vi "Testing Mode.vi"(7 "Filepath":path=path "D:/My Project/2019-2020/Magnetic Mareli UM/MM_UM/Project Setup/data/program seq/Program_280A.bin") -> (1 "Running Model":string)   [LabVIEW 2015]
uses:
  Control Button/Exit.ctl
  Control Button/Start.ctl
  Test  enqueue/AutoTest seq.ctl
  Test  enqueue/Auot Test selection.ctl
  <vilib>/Analysis/baseanly.llb/Mean (DBL).vi
  Galobal variable_TI.vi
  Project Setup/Globle Variable/GR_Servo.vi
  <vilib>/Utility/file.llb/Read Delimited Spreadsheet (string).vi
  <vilib>/Utility/file.llb/Write Delimited Spreadsheet (string).vi
  <vilib>/Analysis/NI_AALBase.lvlib
panel:
  out "Error code":string
  out "Camera Status":T1
  out "x .and. y?":bool
  out "Error":bool
  in  "value":bool
  in  "Tracibility":bool=TRUE
  out "In Range?":bool
  in  "Result":string
  out "Barcode Setting":T2
  in  "Total Counter":string
  out "D.S Tail Tell Barcode":string
  out "D.S Blinker Barcode":string
  out "Dail Speedo Barcode":string
  out "Reset":bool
  out "Emergency":bool
  out "Max Load(N)":string
  out "Min Load(N)":string
  in  "Actual Load(N)":string
  out "Load Cell":dbl format="%0.03f"
  in  "Load Offset":dbl
  out "max value":dbl
  out "Dail RPM Barcode":string
  out "Camera NG_P13":bool
  out "Camera OK_P12":bool
  out "Difusser_AI5":bool
  out "Difusser_AI4":bool
  out "Job ID":string
  in  "Graph Reset":bool
  in  "Safety Enb":bool
  in  "Tab Control":enum32{"Test", "Home call"}(tab)
  in  "test":string[][](table)=[["1", "Light Box Ionization", "Pass"], ["2", "Light box Clamp", "Pass"], ["3", "Difusser Put on Light Box", "Pass"], ["4", "Photo Prism Put On LB", "Test In Progress"], ["5", "LCD Put On Light Box", ""], ["6", "Difusser Checking Position", ""], ["7", "Adesive Tap check Camera", ""], ["8", "LCD Placing Position", ""], ["9", "Camera check Adhesive Taps", ""], ["10", "LCD Display Rotating ", ""], ["11", "Camera Slide Unit", ""], ["12", "LCD Pressing Servo", ""], ["13", "LCD Pressing servo up", ""], ["14", "Camera Unit Rev", ""], ["15", "Fixture Slide Up", ""], ["16", "Light Box Unclamp", ""]]
  in  "Home":string[][](table)
  out "stripped path":path
  in  "Tab":enum32{"Image Display", "Load Graph"}(tab)
  out "2D Picture":picture
  out "Force Vs Time":dbl[](graph)
  in  "String":string
  in  "Vacuum bit":bool
  out "MIC Code":string
  out "Date time":string
  in  "NG Counter":string
  in  "OK Counter":string
  out "User Name":string
  in  "Cycle":i32
  in  "Slide Servo Home Call":bool
  out "D-enqueue":T3
  in  "Home Call":bool
  out "DI":bool[](array[boolean])
  in  "Error Message":string
  out "Current Date & Time":timestamp
  out "Cycle Time(Sec)":i32
  in  "Start":T4
  in  "Cycle Start Bit":bool
  in  "vi reference":refnum<vi>
  in  "Reset Ct.":bool
  out "error out":errorcluster
  in  "Tbl Refnum":refnum<vi>
  in  "Image Display":bool
  in  "Exit":T5
  # "Enable"
  # "Disable"
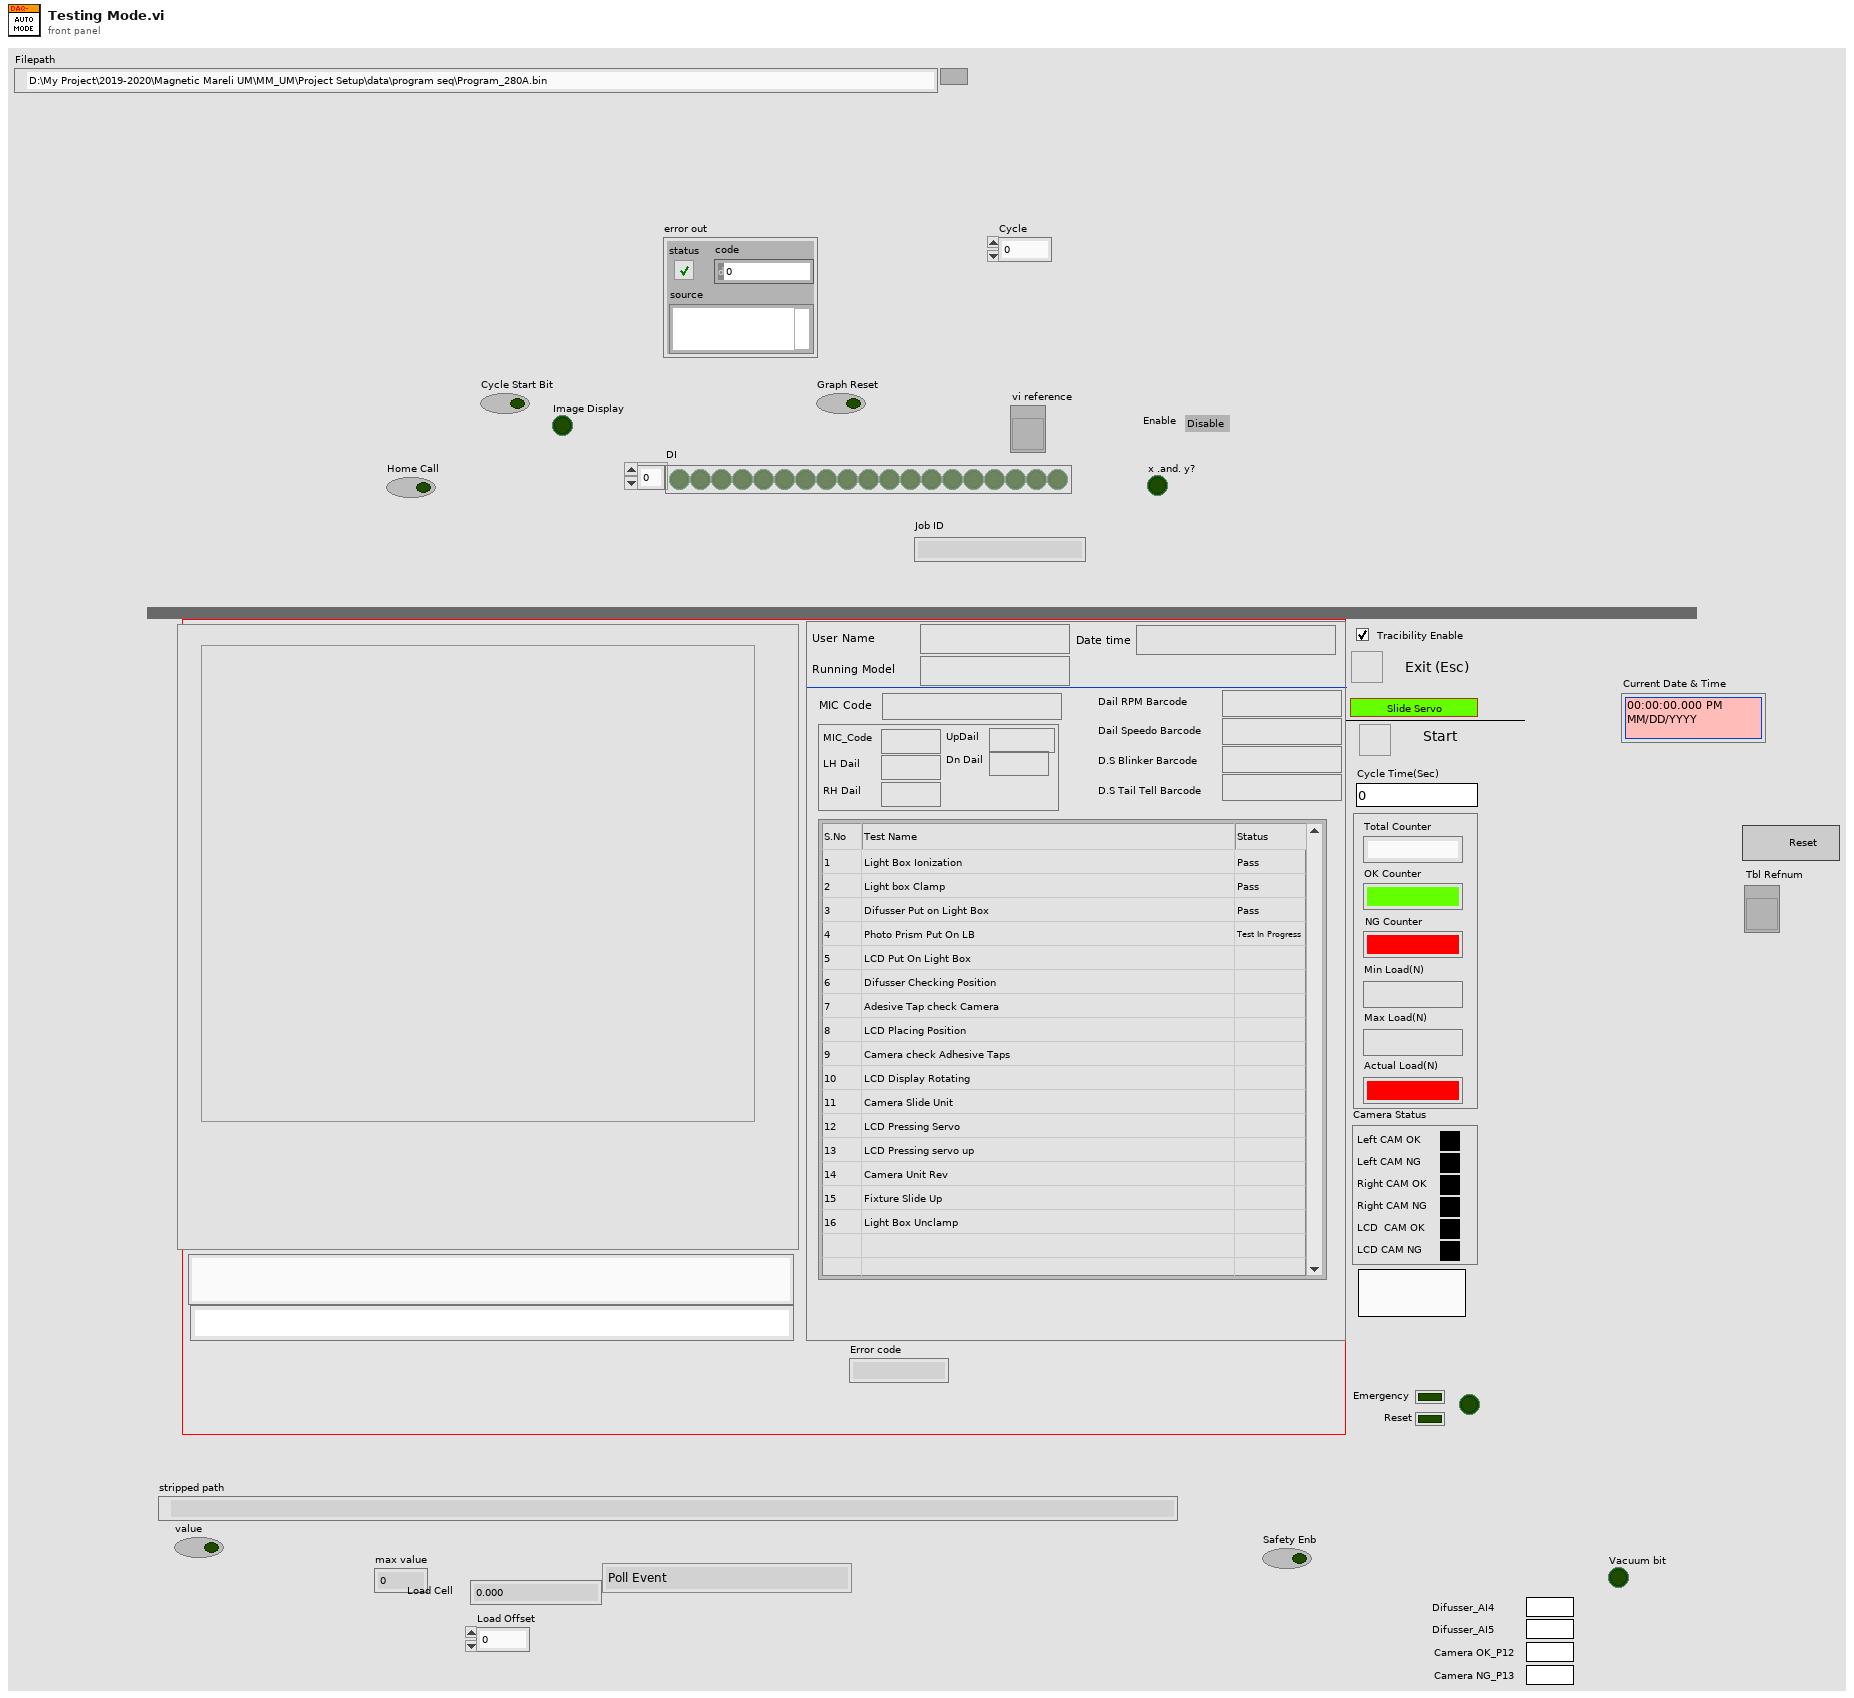
[diagram p1: front panel]
types:
  T1 = cluster{"Left CAM OK":bool, "Left CAM NG":bool, "Right CAM OK":bool, "Right CAM NG":bool, "LCD  CAM OK":bool, "LCD CAM NG ":bool}
  T2 = cluster{"MIC_Code":string, "LH Dail":string, "RH Dail":string, "UpDail":string, "Dn Dail":string}
  T3 = typedef "AutoTest seq.ctl" = enum16{"Poll Event", "Cylender Home ", "Initilization", "Read Barcode", "Slide Servo send Cammand", "Slide Servo Home Call", "Slide Servo Reset", "Camera Co-ordinate_1", "Home Call", "Result Save", "Exit"}
  T4 = typedef "Start.ctl" = bool
  T5 = typedef "Exit.ctl" = bool
  T6 = typedef "Auot Test selection.ctl" = enum16{"Init", "Enqueue ", "Enqueue N", "Enqueue in stack", "Enqueue in stack N", "Dequeue", "Dequeue N", "Flush", "Release Queue"}
  T7 = cluster{"MaxLoad(N) ":dbl, "Min Load(N)":dbl, "Load Offset":dbl, "Model":string, "MIC Code":string, "Dial Speedo":string, "Dial RMP":string, "Blinker":string, "Telltale":string}
  T8 = cluster{"Item Name":string, "Item Status":bool, "Steps":cluster{"Channel Type":string, "Channels":string, "Wait/Poll (ms)":u32, "Parameter":u8, "STM-Speed":i32, "STM-Degree":u32, "Direction":u8}[]}[]
  T9 = cluster{"No. Fail Coun t":string, "Rework Status Count 0\\1":string, "NA Count Max =3 ":string, "Testesd Count  0/1":string, "Error code":string}
  T10 = enum16{"Height Check Cyl up(P0.23_07)", "Height Check Cyl  Up RS_(AI12_26)", "Height Check Cyl  Dn RS_(AI13_27)", "Height Check Cyl dn(P0.24_08)", "Camera Cyl Rev(P0.26_10)", "Camera Cyl fwd(P0.25_09)", "Height Check Cyl off", "Camera Cyl Rev_RS(AI15_29)", "Camera Cyl off", "Camera Cyl FWD_RS(AI14_28)", "LCD Rotation Dn(P0.28_12)", "LCD Rotation dn proxi(AI17_31)", "LCD Rotation Up(P0.27_11)", "LCD Rotation dn proxi(AI16_30)"}
  T11 = cluster{"Start":bool, "Emergency ":bool, "Reset":bool, "Home":bool, "Safety":bool}
  T12 = cluster{"[0]":string, "[1]":string, "[2]":string, "[3]":string, "[4]":string, "[5]":string, "[6]":string, "[7]":string}
  T13 = cluster{"[0]":string, "[1]":string, "[2]":string, "[3]":string, "[4]":string}
  T14 = cluster{"Emergency":bool, "Air Pressure":bool, "Saftey Sensor":bool, "Slide Servo  fault":bool, "Reset":bool, "Pressing Cyl Up RS_AI19":bool}
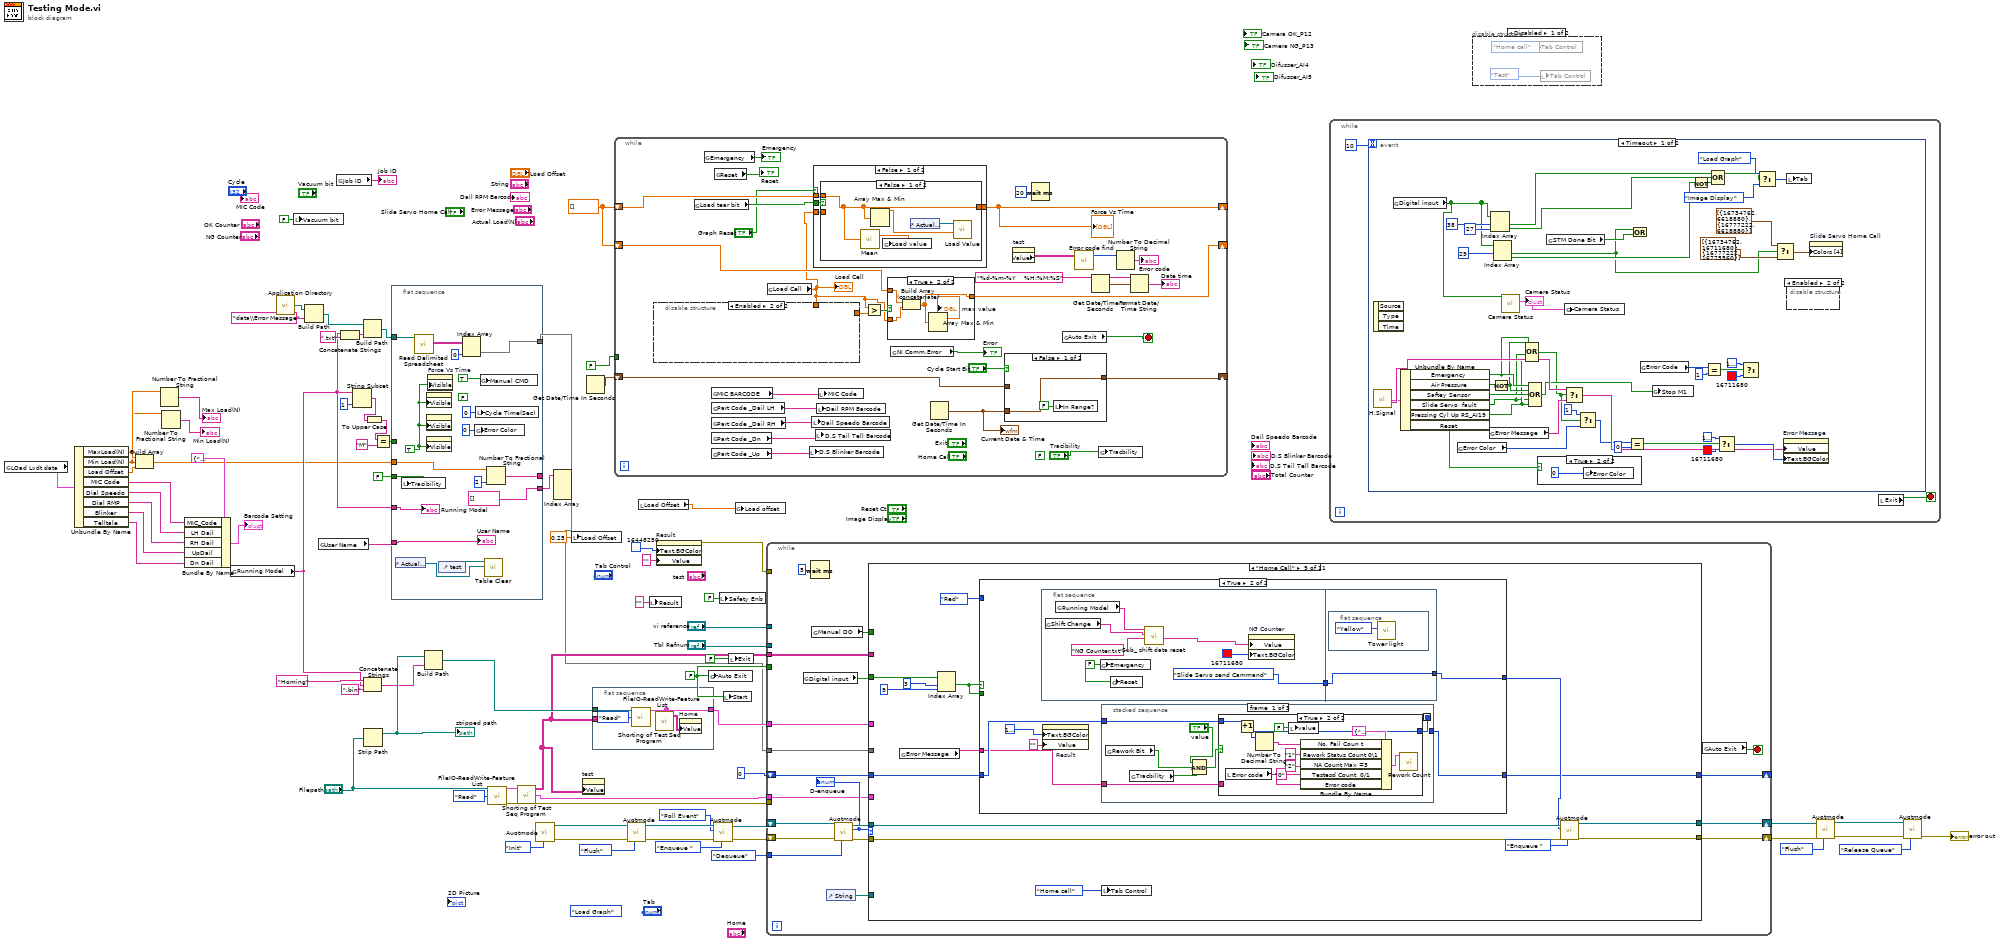
[diagram p0: block diagram]
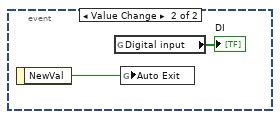
[diagram p5: hidden frame]
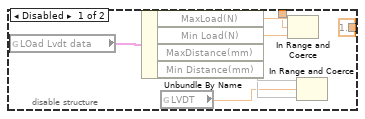
[diagram p6: hidden frame]
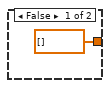
[diagram p7: hidden frame]
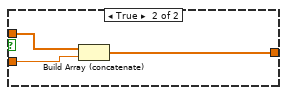
[diagram p8: hidden frame]
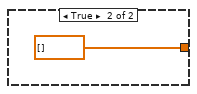
[diagram p9: hidden frame]
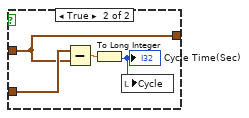
[diagram p10: hidden frame]
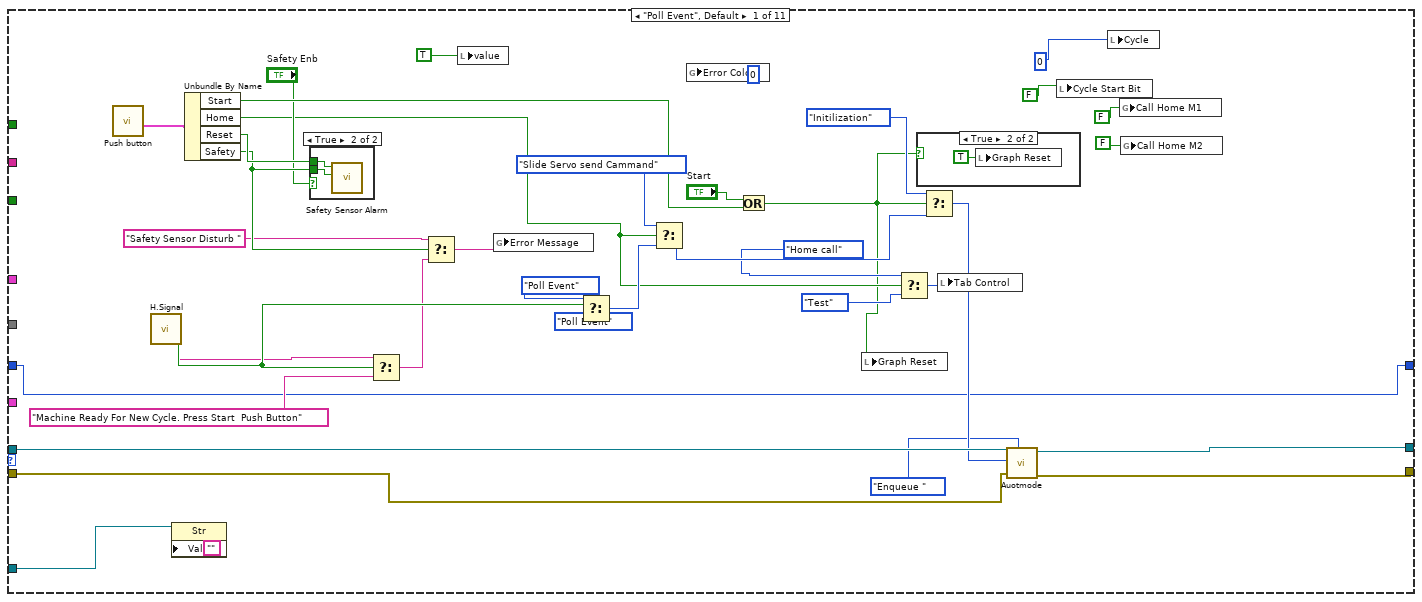
[diagram p11: hidden frame]
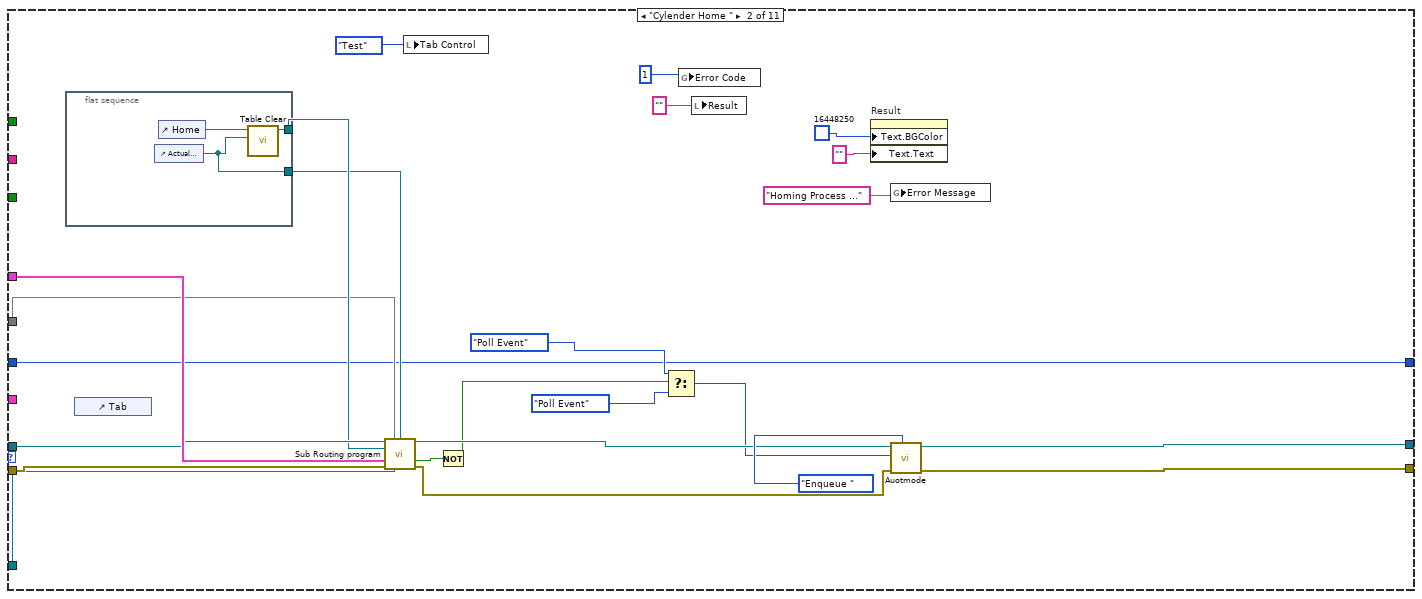
[diagram p14: hidden frame]
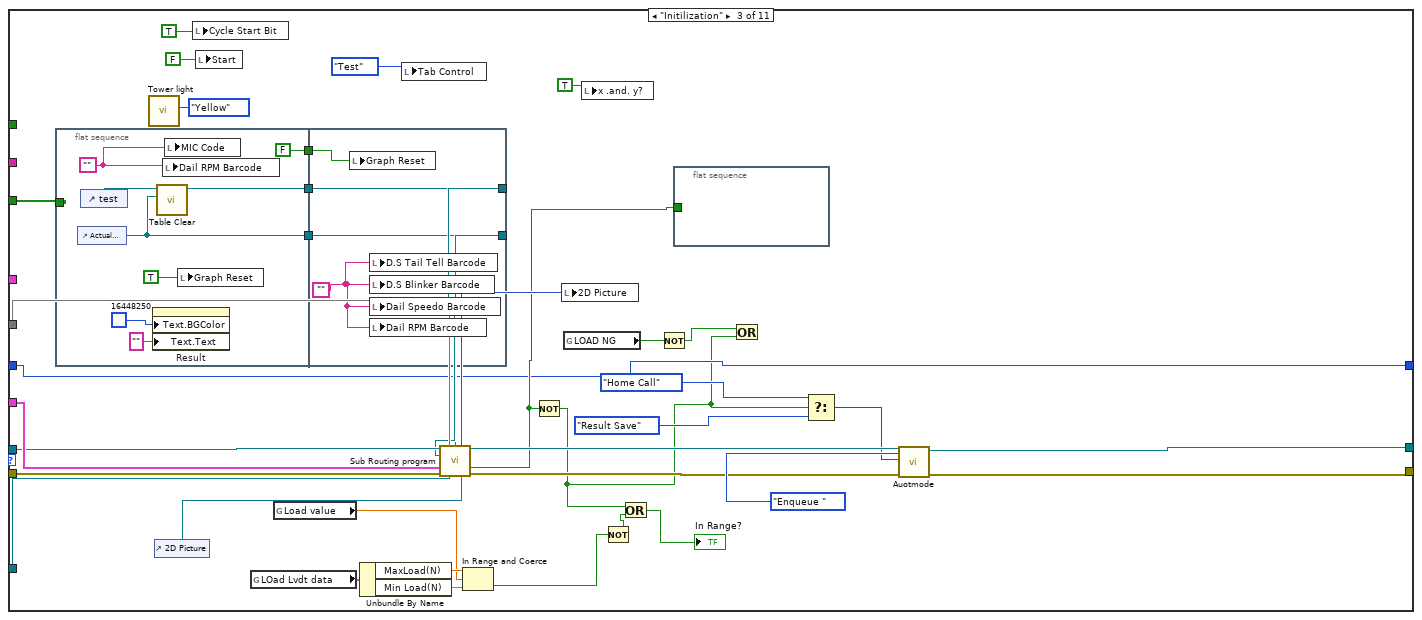
[diagram p15: hidden frame]
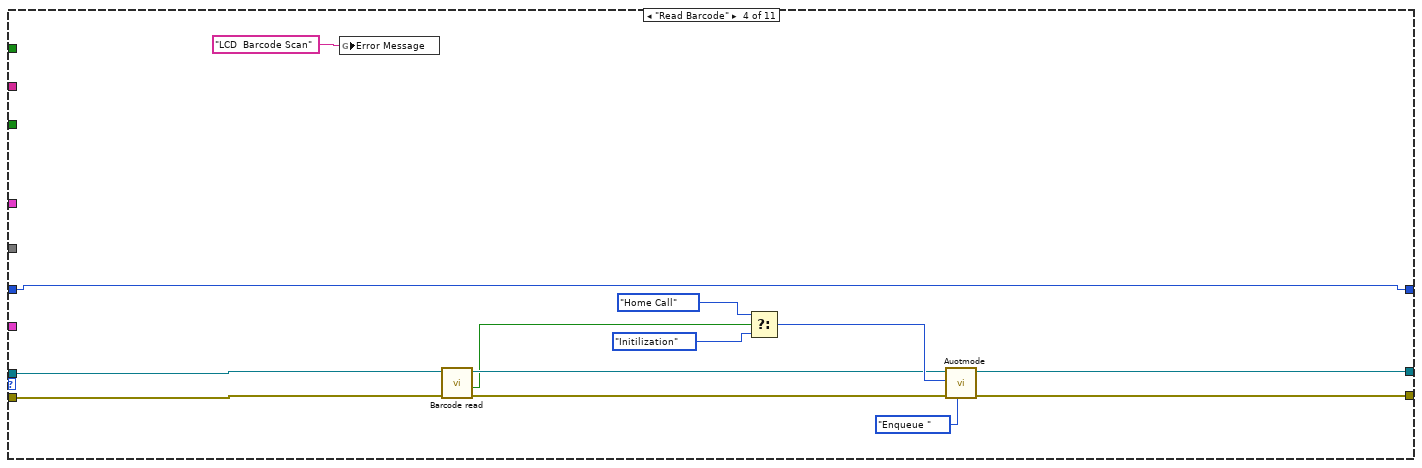
[diagram p16: hidden frame]
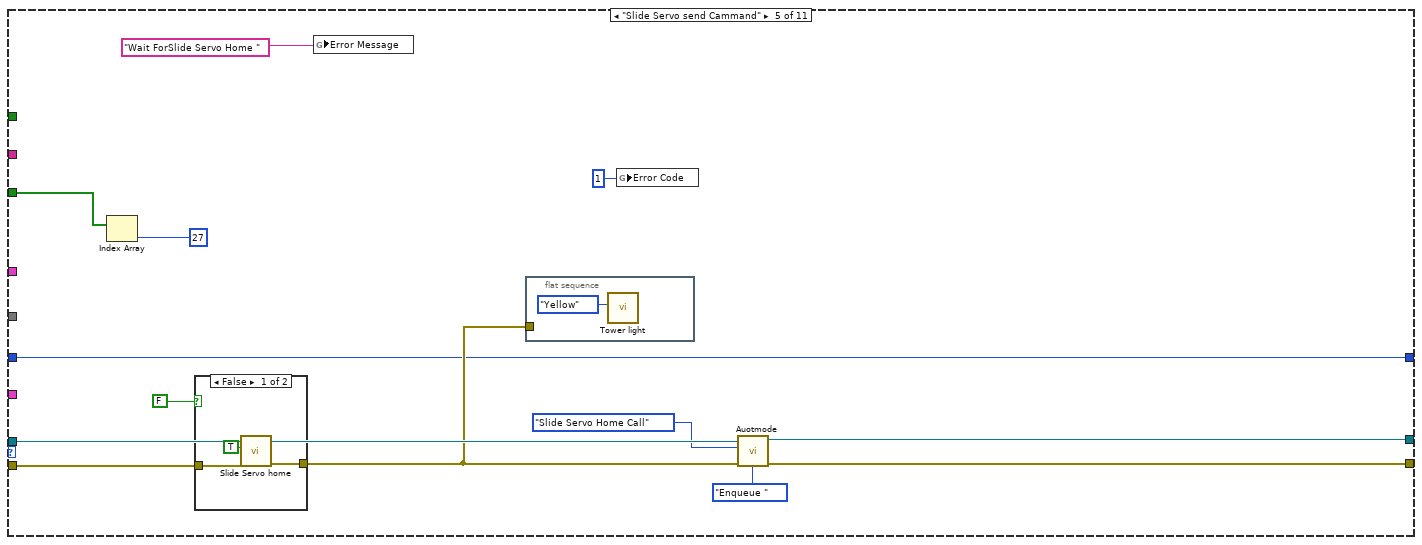
[diagram p17: hidden frame]
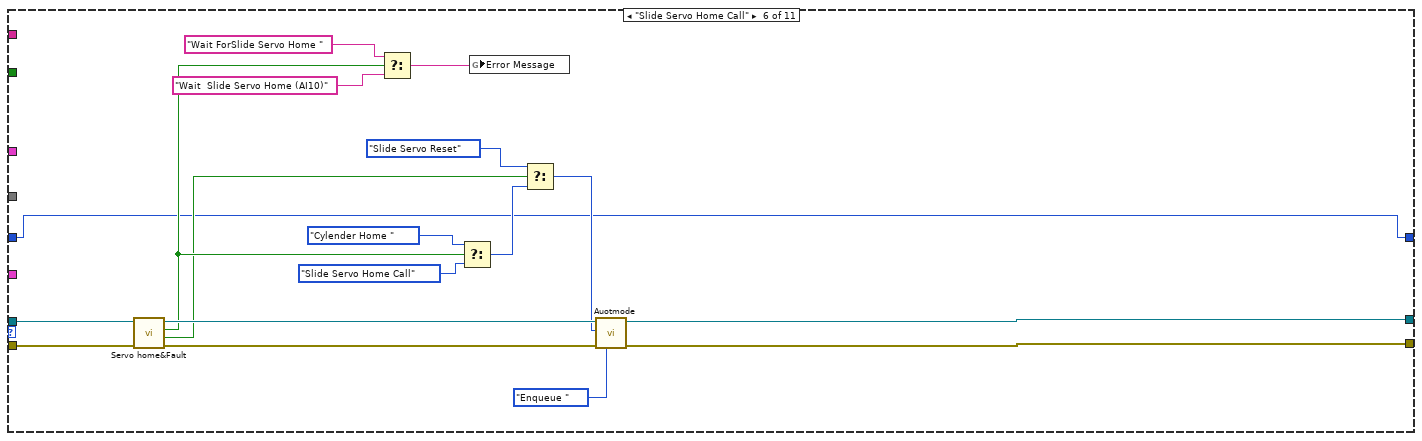
[diagram p19: hidden frame]
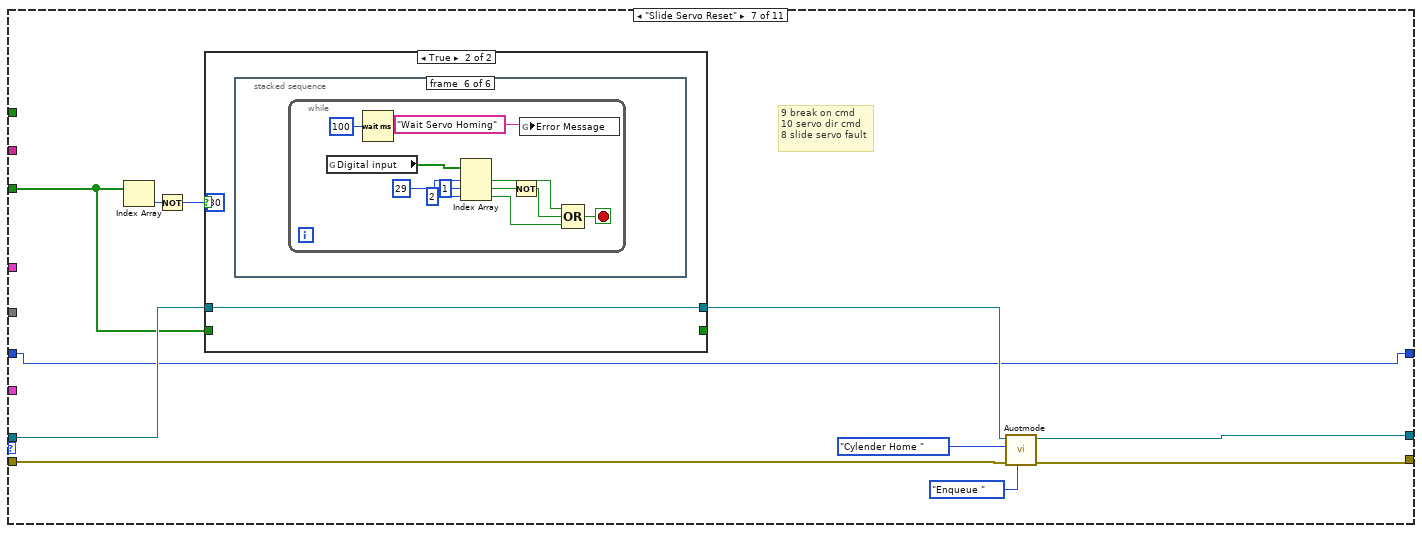
[diagram p20: hidden frame]
diagram:
  (unwired) enum32{"Image Display", "Load Graph"}."Load Graph" ("Tab")
  w41 = dbl[] []
  w53 = FALSE ("Auto Exit")
  n1 = global read "Galobal variable_TI.vi" "LOad Lvdt data"() -> (w22:T7)
  n2 = Unbundle By Name(w22) -> ("MaxLoad(N)"=w8:dbl, "Min Load(N)"=w7:dbl, "Load Offset"=w21:dbl, "MIC Code"=w19:string, "Dial Speedo"=w18:string, "Dial RMP"=w17:string, "Blinker"=w16:string, "Telltale"=w15:string)
  n3 = Build Array(w8, w7, w21) -> (w13:dbl[])
  n4 = Number To Fractional String(number=w8) -> (F-format string=→"Max Load(N)":string)  [unwired: 3 in]
  n5 = Number To Fractional String(number=w7) -> (F-format string=→"Min Load(N)":string)  [unwired: 3 in]
  n6 = Bundle By Name(cluster=T2 {"MIC_Code"="", "LH Dail"="", "RH Dail"="", "UpDail"="", "Dn Dail"=""} ("Barcode Setting"), "MIC_Code"=w19, "LH Dail"=w18, "RH Dail"=w17, "UpDail"=w16, "Dn Dail"=w15) -> (→"Barcode Setting":T2)
  n7 = global read "Galobal variable_TI.vi" "Running Model"() -> (w32:string)
  n8 = call <vilib>:"Application Directory.vi"() -> ("Application Directory"=w37:path)
  n9 = local write "Vacuum bit"(FALSE ("Vacuum bit")) -> ()
  n10 = Build Path(base path=w37, name or relative path="data\\Error Message") -> (appended path=w38:path)
  n11 = global read "Galobal variable_TI.vi" "User Name"() -> (w52:string)
  n12 = global read "Galobal variable_TI.vi" "Job ID"() -> (→"Job ID":string)
  n13 = Concatenate Strings(w32, ".txt" ("string")) -> (w35:string)
  n14 = String Subset(string=w32, length (rest)=1 ("length (rest)")) -> (substring=w27:string)  [unwired: 1 in]
  n15 = Build Path(base path=w38, name or relative path=w35) -> (appended path=w34:path)
  n16 = Concatenate Strings("Homing" ("string"), w32, ".bin" ("string")) -> (w42:string)
  n17 = Strip Path(path="Filepath") -> (stripped path=w49:path)  [unwired: 1 out]
  "stripped path" <- w49
  n18 = To Upper Case(1:w27) -> (0:w30:string)
  n19 = Equal?(x=w30, y="M") -> (x = y?=w28:bool)
  n20 = flat-sequence {
    tunnel: [w92] -> _
    tunnel: w32 -> [w91]
    tunnel: w52 -> [w90]
    tunnel: w34 -> [w87]
    tunnel: [w84] -> w33
    tunnel: w28 -> [_]
    tunnel: [string[] [] ("array")] -> w24
    tunnel: w13 -> [w80]
    tunnel: FALSE -> [w78]
    frame #0 {
      w81 = TRUE
      (unwired) FALSE ("LCD Servo Home Call")
      n21 = control-ref of="Actual Load(N)"() -> (w88:refnum<vi>)
      n22 = local write "Tracibility"(w78) -> ()
      n23 = call-poly <vilib>:"Read Delimited Spreadsheet.vi"("file path (dialog if empty)"=w87) -> ("all rows"=w86:string[][])  [unwired: 9 in, 5 out]
      n24 = property on="Min Load(N)" class="Str"("Visible"=w81) -> ()  [unwired: 2 in, 2 out]
      n25 = property on="Max Load(N)" class="Str"("Visible"=w81) -> ()  [unwired: 2 in, 2 out]
      n26 = property on="Actual Load(N)" class="Str"("Visible"=w81) -> ()  [unwired: 2 in, 2 out]
      n27 = property on="Force Vs Time" class="WFGraph (strict)"("Visible"=w81) -> ()  [unwired: 2 in, 2 out]
      n28 = control-ref of="test"() -> (w89:refnum<vi>)
      n29 = Index Array(array=w86, index (col)=0 ("disabled index (col)")) -> (element=w84:string[])  [unwired: 1 in]
      n30 = global write "GR_Servo.vi" "Error Color"(0 ("Error Color")) -> ()
      n31 = local write "Cycle Time(Sec)"(0 ("Cycle Time(Sec)")) -> ()
      n32 = global write "Galobal variable_TI.vi" "Manual CMD"(TRUE ("Manual CMD")) -> ()
      n33 = call "Table Clear.vi"("Load"=w88, "Table (In)"=w89) -> ()  [unwired: 8 in, 2 out]
      n34 = Number To Fractional String(number=w80, precision (6)=i16 2) -> (F-format string=w92:string[])  [unwired: 2 in]
      "User Name" <- w90
      "Running Model" <- w91
    }
  }
  n35 = Build Path(base path=w49, name or relative path=w42) -> (appended path=w48:path)
  n36 = call "FileIO-ReadWrite-FeatureList.vi"("Filepath"="Filepath", "Read/Write"=enum16{"Read", "Write"}."Read") -> ("Feature List (Out)"=w58:T8, "Error Out"=w59:errorcluster)  [unwired: 12 in]
  n37 = call "Shorting of Test Seq Program.vi"("Feature List (Out)"=w58) -> ("Feature Step Enable"=w54:T8, "Feature Name"=w47:string[][])  [unwired: 3 in]
  n38 = call "Auotmode.vi"("Enum Selection"=Auot_Test_selection."Init") -> ("error out"=w71:errorcluster, "queue Out"=w69:refnum<queue>)  [unwired: 7 in, 1 out]
  n39 = Index Array(array=w24) -> ()  [unwired: 4 in, 4 out]
  n40 = local write "Load Offset"(0.25 ("Load Offset")) -> ()
  n41 = property on="test" class="Tbl (strict)"("Value"=w47) -> ()  [unwired: 2 in, 2 out]
  n42 = Get Date/Time In Seconds() -> (seconds since 1Jan1904=w61:timestamp)
  n43 = flat-sequence {
    tunnel: w48 -> [w98]
    tunnel: w47 -> [_]
    tunnel: [w97] -> w46
    frame #0 {
      n44 = call "FileIO-ReadWrite-FeatureList.vi"("Filepath"=w98, "Read/Write"=enum16{"Read", "Write"}."Read") -> ("Feature List (Out)"=w97:T8)  [unwired: 12 in, 1 out]
      n45 = call "Shorting of Test Seq Program.vi"("Feature List (Out)"=w97) -> ("Feature Name"=w96:string[][])  [unwired: 3 in, 1 out]
      n46 = property on="Home" class="Tbl (strict)"("Value"=w96) -> ()  [unwired: 2 in, 2 out]
    }
  }
  n47 = while {
    shift-right: [w128] -> _
    shift-left: w61 -> [w127]
    tunnel: FALSE ("Servo Stop") -> [_]
    shift-right: [w115] -> _
    shift-left: w41 -> [w117]
    shift-right: [w109] -> _
    shift-left: w41 -> [w111]
    stop <- w125 stop-if-true
    (unwired) FALSE ("Tracibility")
    n48 = global read "Galobal variable_TI.vi" "Load tear bit"() -> (w118:bool)
    n49 = global read "Galobal variable_TI.vi" "Emergency"() -> (→"Emergency":bool)
    n50 = global read "Galobal variable_TI.vi" "MIC BARCODE"() -> (w114:string)
    n51 = global read "Galobal variable_TI.vi" "Part Code _Dail LH"() -> (w106:string)
    n52 = global read "Galobal variable_TI.vi" "Part Code _Dail RH"() -> (w105:string)
    n53 = global read "Galobal variable_TI.vi" "Part Code _Dn"() -> (w103:string)
    n54 = global read "Galobal variable_TI.vi" "Part Code _Up"() -> (w104:string)
    n55 = global read "Galobal variable_TI.vi" "Reset"() -> (→"Reset":bool)
    n56 = global read "Galobal variable_TI.vi" "Load Cell"() -> (w110:dbl)
    "Load Cell" <- w110
    n57 = disable-structure shown="Enabled" {
      disable-tunnel: [1.0 ("y") _] -> w113
      disable-tunnel: w110 -> [w129 _]
      frame Disabled {
        n58 = global read "Galobal variable_TI.vi" "LOad Lvdt data"() -> (w136:T7)
        n59 = Unbundle By Name(w136) -> ("MaxLoad(N)"=w135:dbl, "Min Load(N)"=w134:dbl, "MaxDistance(mm)"=w133, "Min Distance(mm)"=w132)
        n60 = global read "Galobal variable_TI.vi" "LVDT"() -> (w131:dbl)
        n61 = In Range and Coerce(upper limit=w135, x=w129, lower limit=w134) -> ()  [unwired: 2 out]
        n62 = In Range and Coerce(upper limit=w133, x=w131, lower limit=w132) -> ()  [unwired: 2 out]
      }
      frame Enabled {
      }
    }
    n63 = local write "D.S Blinker Barcode"(w104) -> ()
    n64 = local write "Dail Speedo Barcode"(w105) -> ()
    n65 = case shown="False" "Graph Reset" {
      tunnel: w118 -> [w142 _]
      tunnel: w110 -> [w145 _]
      tunnel: [w144 dbl[] []] -> w115
      tunnel: w117 -> [w143 _]
      frame False {
        n66 = case shown="False" w142 {
          tunnel: w145 -> [_ w152]
          tunnel: [w147 w150] -> w144
          tunnel: w143 -> [w147 w151]
          frame False {
            n67 = call-poly <vilib>:"Mean.vi"("X"=w147) -> ("mean"=w146:dbl)  [unwired: 1 out]
            n68 = Array Max & Min(array=w147) -> (max value=w148:dbl)  [unwired: 3 out]
            n69 = global write "Galobal variable_TI.vi" "Load value"(w146) -> ()
            n70 = control-ref of="Actual Load(N)"() -> (w149:refnum<vi>)
            n71 = call "Load Value.vi"("Load Cell"=w148, "String in"=w149) -> ()  [unwired: 9 in]
          }
          frame True {
            n72 = Build Array (concatenate)(w151, w152) -> (w150:dbl[])
          }
        }
      }
      frame True {
      }
    }
    "Force Vs Time" <- w115
    n73 = local write "D.S Tail Tell Barcode"(w103) -> ()
    n74 = local write "Dail RPM Barcode"(w106) -> ()
    n75 = local write "MIC Code"(w114) -> ()
    n76 = Greater?(x=w110, y=w113) -> (0:w112:bool)
    n77 = case shown="True" w112 {
      tunnel: w111 -> [_ w140]
      tunnel: w110 -> [_ w139]
      tunnel: [dbl[] [] w138] -> w109
      frame False {
      }
      frame True {
        n78 = Build Array (concatenate)(w140, w139) -> (w138:dbl[])
        n79 = Array Max & Min(array=w138) -> (max value=→"max value":dbl)  [unwired: 3 out]
      }
    }
    n80 = global read "Galobal variable_TI.vi" "NI Comm.Error"() -> (→"Error":bool)
    n81 = Get Date/Time In Seconds() -> (seconds since 1Jan1904=w124:timestamp)
    "Current Date & Time" <- w124
    n82 = case shown="False" "Cycle Start Bit" {
      tunnel: w127 -> [_ w157]
      tunnel: w124 -> [w155 w158]
      tunnel: [w155 w157] -> w128
      frame False {
        n83 = local write "In Range?"(FALSE ("In Range?")) -> ()
      }
      frame True {
        n84 = Subtract(x=w158, y=w157) -> (x-y=w159:dbl)
        n85 = To Long Integer(number=w159) -> (32bit integer=w156:i32)
        "Cycle Time(Sec)" <- w156
        n86 = local write "Cycle"(w156) -> ()
      }
    }
    n87 = property on="test" class="Tbl (strict)"() -> ("Value"=w101:string[][])  [unwired: 2 in, 2 out]
    n88 = Wait (ms)(milliseconds to wait=u32 20) -> ()  [unwired: 1 out]
    n89 = global read "Galobal variable_TI.vi" "Auto Exit"() -> (w125:bool)
    n90 = call "Error code find.vi"("Table Control"=w101) -> ("Error code"=w100:i32)  [unwired: 2 in]
    n91 = Get Date/Time In Seconds() -> (seconds since 1Jan1904=w122:timestamp)
    n92 = global write "Galobal variable_TI.vi" "Tracbility"("Tracibility") -> ()
    n93 = Number To Decimal String(number=w100) -> (decimal integer string=→"Error code":string)  [unwired: 1 in]
    n94 = Format Date/Time String(time format string (%c)="%d-%m-%Y    %H:%M:%S", seconds (now)=w122) -> (date/time string=→"Date time":string)  [unwired: 1 in]
  }
  n95 = call "Auotmode.vi"("Enum Selection"=Auot_Test_selection."Flush", "Error In"=w71, "queue in"=w69) -> ("error out"=w70:errorcluster, "queue Out"=w68:refnum<queue>)  [unwired: 5 in, 1 out]
  n96 = local read "Load Offset"() -> (w25:dbl)
  n97 = local write "Result"("" ("Result")) -> ()
  n98 = property on="Result" class="Str"("Text.BGColor"=u32 16448250 ("Color Box"), "Value"="" ("Text.Text")) -> (error out=w10:errorcluster)  [unwired: 2 in, 1 out]
  n99 = global write "Galobal variable_TI.vi" "Auto Exit"(w53) -> ()
  n100 = call "Auotmode.vi"("Enum Selection"=Auot_Test_selection."Enqueue ", "Error In"=w70, "Enqueue"=AutoTest_seq."Poll Event", "queue in"=w68) -> ("error out"=w75:errorcluster, "queue Out"=w56:refnum<queue>)  [unwired: 4 in, 1 out]
  n101 = local write "Safety Enb"(FALSE ("Safety Enb")) -> ()
  n102 = local write "Start"(w53) -> ()
  n103 = local write "Exit"(T5 FALSE ("Exit")) -> ()
  n104 = global write "Galobal variable_TI.vi" "Load offset"(w25) -> ()
  n105 = while {
    tunnel: "vi reference" -> [_]
    tunnel: "Tbl Refnum" -> [_]
    tunnel: w54 -> [w171]
    tunnel: w59 -> [_]
    tunnel: w33 -> [w172]
    shift-right: [w175] -> w62
    shift-left: w56 -> [w169]
    shift-right: [w168] -> w2
    shift-left: w75 -> [w177]
    tunnel: w53 -> [_]
    tunnel: w47 -> [w167]
    tunnel: w46 -> [w164]
    tunnel: w10 -> [_]
    shift-right: [w161] -> _
    shift-left: 0 ("index") -> [w162]
    tunnel: Auot_Test_selection."Dequeue" ("Enum Selection") -> [w160]
    stop <- w170 stop-if-true
    n106 = global read "Galobal variable_TI.vi" "Digital input"() -> (w166:bool[])
    n107 = Wait (ms)(milliseconds to wait=u32 5) -> ()  [unwired: 1 out]
    n108 = global read "Galobal variable_TI.vi" "Manual DO"() -> (w165:bool[])
    n109 = control-ref of="String"() -> (w163:refnum<vi>)
    n110 = call "Auotmode.vi"("Enum Selection"=w160, "Error In"=w177, "queue in"=w169) -> ("error out"=w174:errorcluster, "D-enqueue"=w173:T3, "queue Out"=w176:refnum<queue>)  [unwired: 5 in]
    "D-enqueue" <- w173
    n111 = case shown="\"Home Call\"" w173 {
      tunnel: w176 -> [w216 w239 w283 w309 w318 w342 w352 w401 w415 w484 w550]
      tunnel: [w214 w243 w278 w302 w321 w343 w351 w401 w414 w483 w551] -> w175
      tunnel: w174 -> [w215 w237 w282 w308 w319 w341 w348 w400 w413 w482 w553]
      tunnel: [w213 w242 w277 w300 w320 w344 w349 w400 w412 w481 w553] -> w168
      tunnel: w171 -> [_ _ w284 _ _ _ _ _ _ _ _]
      tunnel: w172 -> [_ w234 w274 _ _ _ _ _ _ _ _]
      tunnel: w167 -> [_ _ _ _ _ _ _ _ _ _ _]
      tunnel: w166 -> [_ _ w270 _ w315 _ w346 _ w409 _ _]
      tunnel: w165 -> [_ _ _ _ _ _ _ _ _ _ _]
      tunnel: w164 -> [_ w240 _ _ _ _ _ _ _ _ _]
      tunnel: w163 -> [w198 w228 w267 _ _ _ _ _ _ _ _]
      tunnel: w162 -> [w179 w220 w251 w297 w310 w328 w347 w399 w404 w479 w533]
      tunnel: [w179 w220 w251 w297 w310 w328 w347 w399 w403 w478 w533] -> w161
      frame "Poll Event", Default {
        n112 = call "Push button.vi"() -> ("Push Button"=w200:T11)  [unwired: 9 in, 2 out]
        n113 = call "H.Signal.vi"() -> ("Error Message"=w193:string, "Bool_H Sig"=w194:bool)  [unwired: 12 in, 2 out]
        n114 = property class="Str"(reference=w198, "Value"="") -> ()  [unwired: 1 in, 2 out]
        n115 = Unbundle By Name(w200) -> ("Start"=w199:bool, "Home"=w184:bool, "Reset"=w196:bool, "Safety"=w192:bool)
        n116 = case shown="True" "Safety Enb" {
          tunnel: w196 -> [_ w219]
          tunnel: w192 -> [_ w218]
          frame False {
          }
          frame True {
            n117 = call "Safety Sensor Alarm.vi"("Safety"=w218, "Reset"=w219) -> ()  [unwired: 10 in]
          }
        }
        n118 = Select(t=w193, s=w194, f="Machine Ready For New Cycle. Press Start  Push Button") -> (s? t:f=w190:string)
        n119 = Select(t="Safety Sensor Disturb " ("f"), s=w192, f=w190) -> (s? t:f=w189:string)
        n120 = local write "value"(TRUE ("value")) -> ()
        n121 = global write "GR_Servo.vi" "Error Message"(w189) -> ()
        n122 = Select(t=AutoTest_seq."Poll Event" ("Enqueue"), s=w194, f=AutoTest_seq."Poll Event") -> (s? t:f=w205:T3)
        n123 = Select(t=AutoTest_seq."Slide Servo send Cammand" ("Enqueue"), s=w184, f=w205) -> (s? t:f=w208:T3)
        n124 = global write "GR_Servo.vi" "Error Color"(0 ("Error Color")) -> ()
        n125 = Or(x="Start", y=w199) -> (x .or. y?=w183:T4)
        n126 = local write "Graph Reset"(w183) -> ()
        n127 = Select(t=enum32{"Test", "Home call"}."Home call" ("Tab Control"), s=w184, f=enum32{"Test", "Home call"}."Test" ("Tab Control")) -> (s? t:f=w186:enum32{"Test", "Home call"})
        n128 = case shown="True" w183 {
          frame False {
          }
          frame True {
            n129 = local write "Graph Reset"(TRUE ("Boolean")) -> ()
          }
        }
        n130 = Select(t=AutoTest_seq."Initilization" ("Enqueue"), s=w183, f=w208) -> (s? t:f=w207:T3)
        n131 = local write "Tab Control"(w186) -> ()
        n132 = call "Auotmode.vi"("Enum Selection"=Auot_Test_selection."Enqueue ", "Error In"=w215, "Enqueue"=w207, "queue in"=w216) -> ("error out"=w213:errorcluster, "queue Out"=w214:refnum<queue>)  [unwired: 4 in, 1 out]
        n133 = local write "Cycle Start Bit"(FALSE ("Cycle Start Bit")) -> ()
        n134 = local write "Cycle"(0 ("Cycle")) -> ()
        n135 = global write "Galobal variable_TI.vi" "Call Home M1"(FALSE ("Call Home M1")) -> ()
        n136 = global write "Galobal variable_TI.vi" "Call Home M2"(FALSE ("Call Home M1")) -> ()
      }
      frame "Cylender Home " {
        n137 = flat-sequence {
          tunnel: [w246] -> w235
          tunnel: [w244] -> w227
          frame #0 {
            n138 = control-ref of="Actual Load(N)"() -> (w244:refnum<vi>)
            n139 = control-ref of="Home"() -> (w245:refnum<vi>)
            n140 = call "Table Clear.vi"("Load"=w244, "Table (In)"=w245) -> ("Table (Out)"=w246:refnum<vi>)  [unwired: 8 in, 1 out]
          }
        }
        n141 = control-ref of="Tab"() -> ()  [unwired: 1 out]
        n142 = call "Sub Routing program.vi"("queue Out in"=w239, "FeedBack Channel"=w234, "Load"=w227, "reference in"=w235, "Feature Step Enable"=w240, "error in (no error)"=w237, "Str Refnum"=w228) -> ("Queue out"=w238:refnum<queue>, "Result"=w231:bool, "error out"=w236:errorcluster)  [unwired: 4 in, 2 out]
        n143 = local write "Tab Control"(enum32{"Test", "Home call"}."Test" ("Tab Control")) -> ()
        n144 = Not(x=w231) -> (.not. x?=w230:bool)
        n145 = Select(t=AutoTest_seq."Poll Event" ("Enqueue"), s=w230, f=AutoTest_seq."Poll Event" ("Enqueue")) -> (s? t:f=w229:T3)
        n146 = global write "GR_Servo.vi" "Error Code"(1 ("Error Color")) -> ()
        n147 = local write "Result"("" ("Result")) -> ()
        n148 = property on="Result" class="Str"("Text.BGColor"=u32 16448250 ("Color Box"), "Text.Text"="") -> ()  [unwired: 2 in, 2 out]
        n149 = global write "GR_Servo.vi" "Error Message"("Homing Process ...") -> ()
        n150 = call "Auotmode.vi"("Enum Selection"=Auot_Test_selection."Enqueue ", "Error In"=w236, "Enqueue"=w229, "queue in"=w238) -> ("error out"=w242:errorcluster, "queue Out"=w243:refnum<queue>)  [unwired: 4 in, 1 out]
      }
      frame "Initilization" {
        n151 = flat-sequence {
          tunnel: w270 -> [_]
          tunnel: [w291] -> w261
          tunnel: [w290] -> w260
          tunnel: [FALSE ("Graph Reset")] -> w259
          tunnel: [w295] -> w263
          tunnel: [w296] -> w269
          tunnel: w261 -> [w296]
          tunnel: w260 -> [w295]
          tunnel: w259 -> [w294]
          frame #0 {
            w289 = ""
            n152 = control-ref of="Actual Load(N)"() -> (w290:refnum<vi>)
            n153 = control-ref of="test"() -> (w292:refnum<vi>)
            n154 = property on="Result" class="Str"("Text.BGColor"=u32 16448250 ("Color Box"), "Text.Text"="") -> ()  [unwired: 2 in, 2 out]
            n155 = call "Table Clear.vi"("Load"=w290, "Table (In)"=w292) -> ("Table (Out)"=w291:refnum<vi>)  [unwired: 8 in, 1 out]
            n156 = local write "Dail RPM Barcode"(w289) -> ()
            n157 = local write "MIC Code"(w289) -> ()
            n158 = local write "Graph Reset"(TRUE ("Boolean")) -> ()
          }
          frame #1 {
            w293 = ""
            n159 = local write "Graph Reset"(w294) -> ()
            n160 = local write "D.S Tail Tell Barcode"(w293) -> ()
            n161 = local write "D.S Blinker Barcode"(w293) -> ()
            n162 = local write "Dail Speedo Barcode"(w293) -> ()
            n163 = local write "Dail RPM Barcode"(w293) -> ()
          }
        }
        n164 = call "Tower light.vi"("Enum"=enum16{"Green", "Red", "Yellow"}."Yellow") -> ()  [unwired: 11 in]
        n165 = control-ref of="2D Picture"() -> (w266:refnum<vi>)
        n166 = local write "Cycle Start Bit"(TRUE ("Cycle Start Bit")) -> ()
        n167 = local write "Start"(T4 FALSE ("Start")) -> ()
        n168 = global read "Galobal variable_TI.vi" "LOad Lvdt data"() -> (w255:T7)
        n169 = global read "Galobal variable_TI.vi" "Load value"() -> (w254:dbl)
        n170 = Unbundle By Name(w255) -> ("MaxLoad(N)"=w256:dbl, "Min Load(N)"=w257:dbl)
        n171 = local write "Tab Control"(enum32{"Test", "Home call"}."Test" ("Tab Control")) -> ()
        n172 = call "Sub Routing program.vi"("queue Out in"=w283, "FeedBack Channel"=w274, "Load"=w263, "reference in"=w269, "Feature Step Enable"=w284, "error in (no error)"=w282, "Str Refnum"=w267, "Pict Refnum"=w266) -> ("2D Picture"=w268:picture, "Queue out"=w280:refnum<queue>, "Result"=w262:bool, "error out"=w279:errorcluster)  [unwired: 3 in, 1 out]
        n173 = In Range and Coerce(upper limit=w256, x=w254, lower limit=w257) -> (In Range?=w253:bool)  [unwired: 1 out]
        n174 = Not(x=w262) -> (.not. x?=w247:bool)
        n175 = local write "2D Picture"(w268) -> ()
        n176 = global read "Galobal variable_TI.vi" "LOAD NG"() -> (w249:bool)
        n177 = local write "x .and. y?"(TRUE ("x .and. y?")) -> ()
        n178 = Not(x=w253) -> (.not. x?=w258:bool)
        n179 = Or(x=w247, y=w258) -> (x .or. y?=→"In Range?":bool)
        n180 = Not(x=w249) -> (.not. x?=w248:bool)
        n181 = flat-sequence {
          tunnel: w262 -> [_]
          frame #0 {
          }
        }
        n182 = Or(x=w248, y=w247) -> ()  [unwired: 1 out]
        n183 = Select(t=AutoTest_seq."Home Call" ("Enqueue"), s=w247, f=AutoTest_seq."Result Save" ("Enqueue")) -> (s? t:f=w271:T3)
        n184 = call "Auotmode.vi"("Enum Selection"=Auot_Test_selection."Enqueue ", "Error In"=w279, "Enqueue"=w271, "queue in"=w280) -> ("error out"=w277:errorcluster, "queue Out"=w278:refnum<queue>)  [unwired: 4 in, 1 out]
      }
      frame "Read Barcode" {
        n185 = global write "GR_Servo.vi" "Error Message"("LCD  Barcode Scan") -> ()
        n186 = call "Barcode read.vi"("error in"=w308, "queue in"=w309) -> ("error out"=w301:errorcluster, "exit"=w298:bool, "queue Out 2"=w303:refnum<queue>)  [unwired: 5 in, 2 out]
        n187 = Select(t=AutoTest_seq."Home Call" ("Enqueue"), s=w298, f=AutoTest_seq."Initilization" ("Enqueue")) -> (s? t:f=w307:T3)
        n188 = call "Auotmode.vi"("Enum Selection"=Auot_Test_selection."Enqueue ", "Error In"=w301, "Enqueue"=w307, "queue in"=w303) -> ("error out"=w300:errorcluster, "queue Out"=w302:refnum<queue>)  [unwired: 4 in, 1 out]
      }
      frame "Slide Servo send Cammand" {
        n189 = Index Array(array=w315, index=27) -> ()  [unwired: 1 out]
        n190 = case shown="False" FALSE {
          tunnel: w319 -> [w325 w326]
          tunnel: [w323 w326] -> w316
          frame False {
            n191 = call "Slide Servo home.vi"("error in"=w325, "NewVal"=TRUE) -> ("error out"=w323:errorcluster)  [unwired: 9 in]
          }
          frame True {
          }
        }
        n192 = global write "GR_Servo.vi" "Error Message"("Wait ForSlide Servo Home ") -> ()
        n193 = flat-sequence {
          tunnel: w316 -> [_]
          frame #0 {
            n194 = call "Tower light.vi"("Enum"=enum16{"Green", "Red", "Yellow"}."Yellow") -> ()  [unwired: 11 in]
          }
        }
        n195 = global write "GR_Servo.vi" "Error Code"(1 ("Error Color")) -> ()
        n196 = call "Auotmode.vi"("Enum Selection"=Auot_Test_selection."Enqueue ", "Error In"=w316, "Enqueue"=AutoTest_seq."Slide Servo Home Call", "queue in"=w318) -> ("error out"=w320:errorcluster, "queue Out"=w321:refnum<queue>)  [unwired: 4 in, 1 out]
      }
      frame "Slide Servo Home Call" {
        n197 = call "Servo home&Fault.vi"("error in (no error)"=w341, "Queue in"=w342) -> ("error out"=w339:errorcluster, "Servo Fault"=w332:bool, "Home"=w333:bool, "Queue out"=w340:refnum<queue>)  [unwired: 6 in]
        n198 = Select(t="Wait ForSlide Servo Home ", s=w333, f="Wait  Slide Servo Home (AI10)") -> (s? t:f=w338:string)
        n199 = Select(t=AutoTest_seq."Cylender Home " ("Enqueue"), s=w333, f=AutoTest_seq."Slide Servo Home Call" ("Enqueue")) -> (s? t:f=w331:T3)
        n200 = global write "GR_Servo.vi" "Error Message"(w338) -> ()
        n201 = Select(t=AutoTest_seq."Slide Servo Reset" ("Enqueue"), s=w332, f=w331) -> (s? t:f=w329:T3)
        n202 = call "Auotmode.vi"("Enum Selection"=Auot_Test_selection."Enqueue ", "Error In"=w339, "Enqueue"=w329, "queue in"=w340) -> ("error out"=w344:errorcluster, "queue Out"=w343:refnum<queue>)  [unwired: 4 in, 1 out]
      }
      frame "Slide Servo Reset" {
        # "9 break on cmd\n10 servo dir cmd\n8 slide servo fault"
        n203 = Index Array(array=w346, index=30) -> (element=w356:bool)
        n204 = Not(x=w356) -> (.not. x?=w355:bool)
        n205 = case shown="True" w355 {
          tunnel: [w359 w365] -> w353
          tunnel: w352 -> [w359 w365]
          tunnel: [w358 _] -> _
          tunnel: w346 -> [w358 _]
          frame False {
            n206 = while {
              stop <- w361 stop-if-true
              n207 = global read "Galobal variable_TI.vi" "Digital input"() -> (w362:bool[])
              n208 = Wait (ms)(milliseconds to wait=u32 100) -> ()  [unwired: 1 out]
              n209 = Index Array(array=w362, index=29) -> (element=w361:bool)
              n210 = global write "GR_Servo.vi" "Error Message"("Wait Servo Homing") -> ()
            }
          }
          frame True {
            n211 = stacked-sequence {
              frame #0 {
                n212 = for {
                  N: 20 -> [_]
                  n213 = global read "Galobal variable_TI.vi" "Manual DO"() -> (w373:bool[])
                  n214 = Replace Array Subset(array=w373, new element #1=FALSE ("new element/subarray"), index #1=9 ("index"), new element #2=FALSE ("new element/subarray"), index #2=10 ("index")) -> (w368:bool[])
                  n215 = Wait (ms)(milliseconds to wait=u32 1) -> ()  [unwired: 1 out]
                  n216 = global write "Galobal variable_TI.vi" "Manual DO"(w368) -> ()
                }
              }
              frame #1 {
                n217 = Wait (ms)(milliseconds to wait=u32 200) -> ()  [unwired: 1 out]
              }
              frame #2 {
                n218 = for {
                  N: 20 -> [_]
                  n219 = global read "Galobal variable_TI.vi" "Manual DO"() -> (w380:bool[])
                  n220 = Replace Array Subset(array=w380, new element=TRUE ("new element/subarray"), index=8) -> (w377:bool[])
                  n221 = global write "Galobal variable_TI.vi" "Manual DO"(w377) -> ()
                  n222 = Wait (ms)(milliseconds to wait=u32 1) -> ()  [unwired: 1 out]
                }
              }
              frame #3 {
                n223 = Wait (ms)(milliseconds to wait=u32 200) -> ()  [unwired: 1 out]
              }
              frame #4 {
                n224 = for {
                  N: 20 -> [_]
                  n225 = global read "Galobal variable_TI.vi" "Manual DO"() -> (w387:bool[])
                  n226 = Wait (ms)(milliseconds to wait=u32 1) -> ()  [unwired: 1 out]
                  n227 = Replace Array Subset(array=w387, new element=FALSE ("new element/subarray"), index=8) -> (w384:bool[])
                  n228 = global write "Galobal variable_TI.vi" "Manual DO"(w384) -> ()
                }
              }
              frame #5 {
                n229 = while {
                  stop <- w388 stop-if-true
                  n230 = global read "Galobal variable_TI.vi" "Digital input"() -> (w396:bool[])
                  n231 = Wait (ms)(milliseconds to wait=u32 100) -> ()  [unwired: 1 out]
                  n232 = Index Array(array=w396, index #1=29 ("index"), index #2=1 ("index"), index #3=2 ("index")) -> (element #1=w391:bool, element #2=w392:bool, element #3=w389:bool)
                  n233 = Not(x=w392) -> (.not. x?=w390:bool)
                  n234 = global write "GR_Servo.vi" "Error Message"("Wait Servo Homing") -> ()
                  n235 = Compound Arithmetic op=OR(w391, w390, w389) -> (w388:bool)
                }
              }
            }
          }
        }
        n236 = call "Auotmode.vi"("Enum Selection"=Auot_Test_selection."Enqueue ", "Error In"=w348, "Enqueue"=AutoTest_seq."Cylender Home ", "queue in"=w353) -> ("error out"=w349:errorcluster, "queue Out"=w351:refnum<queue>)  [unwired: 4 in, 1 out]
      }
      frame "Camera Co-ordinate_1" {
      }
      frame "Home Call" {
        n237 = global read "GR_Servo.vi" "Error Message"() -> (w405:string)
        n238 = Index Array(array=w409, index #1=3 ("index"), index #2=9 ("index")) -> (element #1=w402:bool)  [unwired: 1 out]
        n239 = case shown="True" w402 {
          tunnel: [w428 w447] -> w408
          tunnel: enum16{"Green", "Red", "Yellow"}."Red" ("Enum") -> [w431 _]
          tunnel: w405 -> [w425 w443]
          tunnel: w404 -> [w426 w445]
          tunnel: [w426 w444] -> w403
          tunnel: w402 -> [w424 _]
          frame False {
            n240 = call "Tower light.vi"("Enum"=w431) -> ()  [unwired: 11 in]
            n241 = local read "x .and. y?"() -> (w422:bool)
            n242 = Not(x=w424) -> (.not. x?=w423:bool)
            n243 = global write "GR_Servo.vi" "Error Code"(1 ("Error Color")) -> ()
            n244 = And(x=w422, y=w423) -> (x .and. y?=w419:bool)
            n245 = Select(t=AutoTest_seq."Slide Servo send Cammand" ("Enqueue"), s=w424, f=AutoTest_seq."Home Call") -> (s? t:f=w428:T3)
            n246 = Concatenate Strings(w425, "(Press the Home Push Button)") -> (w420:string)
            n247 = case shown="True" w419 {
              tunnel: w420 -> [_ w432]
              frame False {
              }
              frame True {
                n248 = disable-structure shown="Enabled" {
                  disable-tunnel: w432 -> [_ w439]
                  frame Disabled {
                    w433 = u32 16711680 ("Color Box")
                    n249 = global read "Galobal variable_TI.vi" "Running Model"() -> (w435:string)
                    n250 = call "Working Shift Change(A-B &C).vi"() -> ("Shift Change"=w438:string)  [unwired: 9 in]
                    n251 = call "Sub_ shift data reset.vi"("Serial no"="OK Counter.txt" ("File Name"), "Shift"=w438, "Model"=w435) -> ("Serial no"=w436:string)  [unwired: 6 in, 1 out]
                    n252 = property on="NG Counter" class="Str"("Value"=w436, "Text.BGColor"=w433) -> ()  [unwired: 2 in, 2 out]
                    n253 = property on="Result" class="Str"("Text.BGColor"=w433, "Value"="FAIL" ("Text.Text")) -> ()  [unwired: 2 in, 2 out]
                  }
                  frame Enabled {
                    n254 = global write "GR_Servo.vi" "Error Message"(w439) -> ()
                    n255 = local write "x .and. y?"(FALSE ("x .and. y?")) -> ()
                  }
                }
              }
            }
            n256 = property on="Result" class="Str"("Text.BGColor"=u32 16711680, "Value"="Fail" ("Text.Text")) -> ()  [unwired: 2 in, 2 out]
          }
          frame True {
            n257 = flat-sequence {
              tunnel: [AutoTest_seq."Slide Servo send Cammand" ("Enqueue")] -> w446
              tunnel: [w476] -> w447
              tunnel: w446 -> [w476]
              frame #0 {
                w472 = FALSE ("Emergency")
                n258 = global read "Galobal variable_TI.vi" "Shift Change"() -> (w470:string)
                n259 = global read "Galobal variable_TI.vi" "Running Model"() -> (w471:string)
                n260 = global write "Galobal variable_TI.vi" "Emergency"(w472) -> ()
                n261 = global write "Galobal variable_TI.vi" "Reset"(w472) -> ()
                n262 = call "Sub_ shift data reset.vi"("Serial no"="NG Counter.txt" ("File Name"), "Shift"=w470, "Model"=w471) -> ("Serial no"=w469:string)  [unwired: 6 in, 1 out]
                n263 = property on="NG Counter" class="Str"("Value"=w469, "Text.BGColor"=u32 16711680 ("Color Box")) -> ()  [unwired: 2 in, 2 out]
              }
              frame #1 {
                n264 = flat-sequence {
                  frame #0 {
                    n265 = call "Tower light.vi"("Enum"=enum16{"Green", "Red", "Yellow"}."Yellow") -> ()  [unwired: 11 in]
                  }
                }
              }
            }
            n266 = property on="Result" class="Str"("Text.BGColor"=u32 16777225, "Value"="" ("Text.Text")) -> ()  [unwired: 2 in, 2 out]
            n267 = stacked-sequence {
              seq-local: [w449 _ _] -> [_ _ w467]
              tunnel: w445 -> [w450 _ _]
              tunnel: [_ _ w467] -> w444
              tunnel: w443 -> [w448 _ _]
              frame #0 {
                n268 = global read "Galobal variable_TI.vi" "Rework Bit"() -> (w453:bool)
                n269 = global read "Galobal variable_TI.vi" "Tracbility"() -> (w454:bool)
                n270 = Compound Arithmetic op=AND("value", w453, w454) -> (w452:bool)
                n271 = case shown="True" w452 {
                  tunnel: w450 -> [w455 w462]
                  tunnel: [w455 w460] -> w449
                  tunnel: w448 -> [_ _]
                  frame False {
                  }
                  frame True {
                    n272 = local read "Error code"() -> (w456:string)
                    n273 = Increment(x=w462) -> (x+1=w460:i32)
                    n274 = Number To Decimal String(number=w460) -> (decimal integer string=w461:string)  [unwired: 1 in]
                    n275 = local write "value"(FALSE ("value")) -> ()
                    n276 = Bundle By Name(cluster=T9 {"No. Fail Coun t"="", "Rework Status Count 0\\1"="", "NA Count Max =3 "="", "Testesd Count  0/1"="", "Error code"=""} ("Count For Rework"), "No. Fail Coun t"=w461, "Rework Status Count 0\\1"="1" ("Rework Status Count 0\\1"), "NA Count Max =3"="2", "Testesd Count  0/1"="0", "Error code"=w456) -> (w464:T9)
                    n277 = call "Rework Count.vi"("Count For Rework"=w464) -> ()  [unwired: 9 in, 2 out]
                  }
                }
              }
              frame #1 {
                n278 = Wait (ms)(milliseconds to wait=u32 200) -> ()  [unwired: 1 out]
              }
              frame #2 {
                n279 = disable-structure shown="Disabled" {
                  frame Disabled {
                    n280 = global read "Galobal variable_TI.vi" "LOAD NG"() -> ()  [unwired: 1 out]
                  }
                  frame Enabled {
                  }
                }
                n281 = global write "Galobal variable_TI.vi" "RPT Write"(TRUE ("RPT Write")) -> ()
              }
            }
          }
        }
        n282 = local write "Tab Control"(enum32{"Test", "Home call"}."Home call" ("Tab Control")) -> ()
        n283 = call "Auotmode.vi"("Enum Selection"=Auot_Test_selection."Enqueue ", "Error In"=w413, "Enqueue"=w408, "queue in"=w415) -> ("error out"=w412:errorcluster, "queue Out"=w414:refnum<queue>)  [unwired: 4 in, 1 out]
      }
      frame "Result Save" {
        n284 = stacked-sequence {
          frame #0 {
            w504 = u32 6618880 ("Color Box")
            n285 = global write "Galobal variable_TI.vi" "Pokayoka Status"(TRUE ("RPT Write")) -> ()
            n286 = global read "Galobal variable_TI.vi" "Shift Change"() -> (w501:string)
            n287 = disable-structure shown="Disabled" {
              frame Disabled {
                n288 = call "Serial no.vi"() -> ()  [unwired: 11 in, 1 out]
              }
              frame Enabled {
              }
            }
            n289 = global read "Galobal variable_TI.vi" "Running Model"() -> (w505:string)
            n290 = call "Sub_ shift data reset.vi"("Serial no"="OK Counter.txt" ("File Name"), "Shift"=w501, "Model"=w505) -> ("Serial no"=w506:string)  [unwired: 6 in, 1 out]
            n291 = property on="OK Counter" class="Str"("Value"=w506, "Text.BGColor"=w504) -> ()  [unwired: 2 in, 2 out]
            n292 = property on="Result" class="Str"("Text.BGColor"=w504, "Value"="PASS" ("Text.Text")) -> ()  [unwired: 2 in, 2 out]
          }
          frame #1 {
            n293 = call "Tower light.vi"("Enum"=enum16{"Green", "Red", "Yellow"}."Green") -> ()  [unwired: 11 in]
          }
          frame #2 {
            (unwired) AutoTest_seq."Poll Event" ("Enqueue")
            n294 = local read "Min Load(N)"() -> (w527:string)
            n295 = local read "Max Load(N)"() -> (w526:string)
            n296 = local read "Actual Load(N)"() -> (w509:string)
            n297 = local read "Dail RPM Barcode"() -> (w511:string)
            n298 = global read "Galobal variable_TI.vi" "Running Model"() -> (w530:string)
            n299 = Build Array(w527, w526, w509, "" ("element"), w509) -> (w525:string[])
            n300 = local read "Date time"() -> (w532:string)
            n301 = global read "Galobal variable_TI.vi" "User Name"() -> (w531:string)
            n302 = local read "MIC Code"() -> (w512:string)
            n303 = disable-structure shown="Disabled" {
              frame Disabled {
                n304 = global read "Galobal variable_TI.vi" "Load Cell"() -> ()  [unwired: 1 out]
              }
              frame Enabled {
              }
            }
            n305 = Array To Cluster(array=w525) -> (cluster=w524:T12)
            n306 = local read "test"() -> (w513:string[][])
            n307 = Build Array(w532, w531, w530, w511, w512) -> (w529:string[])
            n308 = Array To Cluster(array=w529) -> (cluster=w528:T13)
            n309 = call <vilib>:"Application Directory.vi"() -> ("Application Directory"=w522:path)
            n310 = call "Report Raw Data.vi"("Data"=w528, "Sensor Data"=w524, "test"=w513) -> ("Data"=w516:string[], "Header"=w519:string[])  [unwired: 7 in]
            n311 = Build Path(base path=w522, name or relative path="data\\Report") -> (appended path=w523:path)
            n312 = call "Header Create.vi"("Report Header"=w519, "File Name"="Test Report", "path File"=w523) -> ("error out"=w517:errorcluster, "dup path"=w518:path)  [unwired: 7 in]
            n313 = call-poly <vilib>:"Write Delimited Spreadsheet.vi"("file path (dialog if empty)"=w518, "1D data"=w516, "append to file? (F)"=TRUE, "error in (no error)"=w517, "delimiter (\\t)"="," ("delimiter (\\t)")) -> ()  [unwired: 9 in, 2 out]
          }
        }
        n314 = stacked-sequence {
          tunnel: w479 -> [w485 _ _]
          tunnel: [_ _ 0] -> w478
          frame #0 {
            n315 = global read "Galobal variable_TI.vi" "Rework Bit"() -> (w487:bool)
            n316 = global read "Galobal variable_TI.vi" "Tracbility"() -> (w488:bool)
            n317 = Compound Arithmetic op=AND(w487, w488) -> (w486:bool)
            n318 = case shown="False" w486 {
              tunnel: w485 -> [w489 w495]
              tunnel: [w489 w495] -> _
              frame False {
              }
              frame True {
                n319 = Number To Decimal String(number=w495) -> (decimal integer string=w494:string)  [unwired: 1 in]
                n320 = Bundle By Name(cluster=T9 {"No. Fail Coun t"="", "Rework Status Count 0\\1"="", "NA Count Max =3 "="", "Testesd Count  0/1"="", "Error code"=""} ("Count For Rework"), "No. Fail Coun t"=w494, "Rework Status Count 0\\1"="0" ("Rework Status Count 0\\1"), "NA Count Max =3"="2", "Testesd Count  0/1"="1", "Error code"="No Error") -> (w496:T9)
                n321 = call "Rework Count.vi"("Count For Rework"=w496) -> ()  [unwired: 9 in, 2 out]
              }
            }
          }
          frame #1 {
            n322 = Wait (ms)(milliseconds to wait=u32 200) -> ()  [unwired: 1 out]
          }
          frame #2 {
            n323 = global write "Galobal variable_TI.vi" "RPT Write"(TRUE ("RPT Write")) -> ()
          }
        }
        n324 = call "Auotmode.vi"("Enum Selection"=Auot_Test_selection."Enqueue ", "Error In"=w482, "queue in"=w484) -> ("error out"=w481:errorcluster, "queue Out"=w483:refnum<queue>)  [unwired: 5 in, 1 out]
      }
      frame "Exit" {
        n325 = global read "Galobal variable_TI.vi" "Digital input"() -> (w548:bool[])
        n326 = stacked-sequence {
          tunnel: T10."LCD Rotation Up(P0.27_11)" ("Enum") -> [w554 _ _ _]
          frame #0 {
            n327 = call "Home Call Cylender.vi"("Enum"=w554) -> ()  [unwired: 11 in]
          }
          frame #1 {
            n328 = Wait (ms)(milliseconds to wait=u32 100) -> ()  [unwired: 1 out]
          }
          frame #2 {
            n329 = global read "Galobal variable_TI.vi" "Manual DO"() -> (w557:bool[])
            n330 = Replace Array Subset(array=w557, new element #1=FALSE ("new element/subarray"), index #1=13 ("index"), new element #2=TRUE ("new element/subarray"), index #2=14 ("index")) -> (w556:bool[])
            n331 = global write "Galobal variable_TI.vi" "Manual DO"(w556) -> ()
          }
          frame #3 {
            n332 = Wait (ms)(milliseconds to wait=u32 100) -> ()  [unwired: 1 out]
          }
        }
        n333 = Index Array(array=w548, index #1=30 ("index"), index #2=33 ("index"), index #3=2 ("index")) -> (element #1=w542:bool, element #2=w541:bool, element #3=w538:bool)
        n334 = global write "GR_Servo.vi" "Error Message"("Wait  LCD Display Unit _AI17") -> ()
        n335 = And(x=w542, y=w541) -> (x .and. y?=w540:bool)
        n336 = global write "GR_Servo.vi" "Error Color"(1 ("Error Color")) -> ()
        n337 = Select(t=AutoTest_seq."Poll Event" ("Enqueue"), s=w540, f=AutoTest_seq."Exit" ("Enqueue")) -> (s? t:f=w536:T3)
        n338 = Select(t=AutoTest_seq."Poll Event" ("Enqueue"), s=w538, f=w536) -> (s? t:f=w535:T3)
        n339 = call "Auotmode.vi"("Enum Selection"=Auot_Test_selection."Enqueue ", "Enqueue"=w535, "queue in"=w550) -> ("queue Out"=w551:refnum<queue>)  [unwired: 5 in, 2 out]
      }
    }
    n340 = global read "Galobal variable_TI.vi" "Auto Exit"() -> (w170:bool)
  }
  n341 = while {
    stop <- w564 stop-if-true
    n342 = event shown="[0] Timeout" {
      selector: _ -> [_ _]
      dyn-events: _ -> [_ _]
      timeout: 10 -> [_ _]
      event Timeout {
        n343 = event-data() -> ()  [unwired: 1 in, 3 out]
        n344 = call "H.Signal.vi"() -> ("output cluster"=w568:T14, "Error Message"=w591:string)  [unwired: 12 in, 2 out]
        n345 = global read "Galobal variable_TI.vi" "Digital input"() -> (w567:bool[])
        n346 = Unbundle By Name(w568) -> ("Emergency"=w585:bool, "Air Pressure"=w594:bool, "Saftey Sensor"=w593:bool, "Slide Servo  fault"=w571:bool, "Pressing Cyl Up RS_AI19"=w583:bool, "Reset"=w570:bool)
        n347 = global read "GR_Servo.vi" "Error Color"() -> (w589:i32)
        n348 = global read "GR_Servo.vi" "Error Message"() -> (w592:string)
        n349 = Index Array(array=w567, index #1=38 ("index"), index #2=27 ("index")) -> (element #1=w565:bool, element #2=w577:bool)
        n350 = Not(x=w594) -> (.not. x?=w584:bool)
        n351 = Index Array(array=w567, index #1=29 ("index")) -> (element #1=w572:bool, element #2=w580:bool)  [unwired: 1 in]
        n352 = call "Camera Status.vi"("Digital input"=w567) -> ("Camera Status"=w566:T1)  [unwired: 10 in]
        "Camera Status" <- w566
        n353 = Compound Arithmetic op=OR(w585, w584, w571, w583) -> (w581:bool)
        n354 = Compound Arithmetic op=OR(w585, w584, w593, w571, w583) -> (w582:bool)
        n355 = case shown="True" w570 {
          frame False {
          }
          frame True {
            n356 = global write "GR_Servo.vi" "Error Color"(0 ("y")) -> ()
          }
        }
        n357 = global read "Galobal variable_TI.vi" "STM Done Bit"() -> (w606:bool)
        n358 = global write "Galobal variable_TI.vi" "Camera Status"(w566) -> ()
        n359 = Select(t=w591, s=w581, f=w592) -> (s? t:f=w590:string)
        n360 = Select(t=1 ("y"), s=w581, f=w589) -> (s? t:f=w587:i32)
        n361 = Equal?(x=w587, y=0) -> (x = y?=w602:bool)
        n362 = Or(x=w572, y=w606) -> ()  [unwired: 1 out]
        n363 = global read "GR_Servo.vi" "Error Code"() -> (w569:i32)
        n364 = global write "Galobal variable_TI.vi" "Stop M1"(w582) -> ()
        n365 = Not(x=w580) -> (.not. x?=w573:bool)
        n366 = Equal?(x=w569, y=1) -> (x = y?=w598:bool)
        n367 = Compound Arithmetic op=OR(w565, w577, w573) -> ()  [unwired: 1 out]
        n368 = Select(t=u32 16777226 ("Color Box"), s=w602, f=u32 16711680 ("Color Box")) -> (s? t:f=w599:u32)
        n369 = Select(t=u32 16777226 ("Color Box"), s=w598, f=u32 16711680 ("Color Box")) -> ()  [unwired: 1 out]
        n370 = Select(t=enum32{"Image Display", "Load Graph"}."Load Graph" ("Tab"), s=w565, f=enum32{"Image Display", "Load Graph"}."Image Display" ("Tab")) -> (s? t:f=w574:enum32{"Image Display", "Load Graph"})
        n371 = Select(t=cluster{u32, u32}[] [{16734762, 6618880}, {16777222, 6618880}] ("Colors [4]"), s=w572, f=cluster{u32, u32}[] [{16734762, 16711680}, {16777222, 16775560}] ("Colors [4]")) -> (s? t:f=w607:cluster{u32, u32}[])
        n372 = property on="Error Message" class="Str"("Value"=w590, "Text.BGColor"=w599) -> ()  [unwired: 2 in, 2 out]
        n373 = local write "Tab"(w574) -> ()
        n374 = disable-structure shown="Enabled" {
          frame Disabled {
          }
          frame Enabled {
          }
        }
        n375 = property on="Slide Servo Home Call" class="Bool (strict)"("Colors [4]"=w607) -> ()  [unwired: 2 in, 2 out]
      }
      event Value Change {
        n376 = event-data() -> ("NewVal"=w609:T5)  [unwired: 1 in]
        n377 = global read "Galobal variable_TI.vi" "Digital input"() -> (→"DI":bool[])
        n378 = global write "Galobal variable_TI.vi" "Auto Exit"(w609) -> ()
      }
    }
    n379 = local read "Exit"() -> (w564:T5)
  }
  n380 = disable-structure shown="Disabled" {
    frame Disabled {
      n381 = local write "Tab Control"(enum32{"Test", "Home call"}."Home call" ("Tab Control")) -> ()
      n382 = local write "Tab Control"(enum32{"Test", "Home call"}."Test" ("Tab Control")) -> ()
    }
    frame Enabled {
    }
  }
  n383 = call "Auotmode.vi"("Enum Selection"=Auot_Test_selection."Flush", "Error In"=w2, "queue in"=w62) -> ("error out"=w67:errorcluster, "queue Out"=w66:refnum<queue>)  [unwired: 5 in, 1 out]
  n384 = call "Auotmode.vi"("Enum Selection"=Auot_Test_selection."Release Queue", "Error In"=w67, "queue in"=w66) -> ("error out"=→"error out":errorcluster)  [unwired: 5 in, 2 out]
